vi "BRig_dataBlock_nReward.vi"() -> (2 "output_nReward":i32)   [LabVIEW 2014]
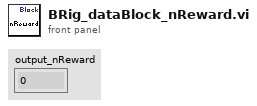
[diagram p1: front panel]
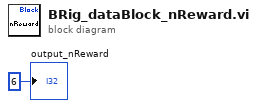
[diagram p0: block diagram]
diagram:
  "output_nReward" <- 6 ("output_iBlock")
